vi "MESS压力值上传测试.vi"(8 "error in (no error)":errorcluster caption="错误输入（无错误）", 9 "barcode":string="C0C50E0004010", 10 "accessKey":string="a45b2d3334ffs_", 11 "Url":string="http://10.6.1.31:8080/MesInnerpackLineIO.asmx") -> (0 "error out":errorcluster caption="错误输出", 3 "ValidateBarcode":string="True,10270194,C.0C.50E,Firehawk药物支架系统（CE无标签）RV3035,RV3035,10")   [LabVIEW 2017]
uses:
  D:/Inspect System/Source Code/Andafa.IO.Helper.dll
  Andafa.IO.Helper.dll
panel:
  # "http://10.6.1.31:8080/MesInnerpackLineIO.asmx"
  # "a45b2d3334ffs_"
  # "C0C50E0004010"
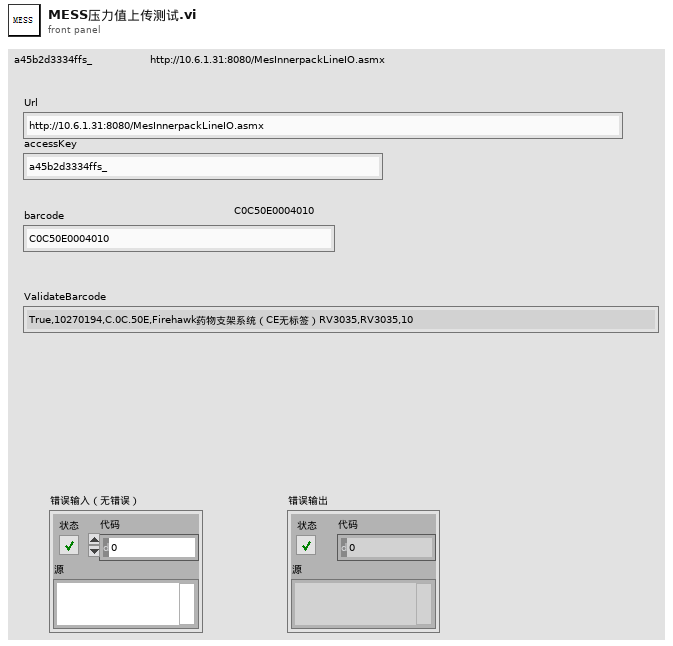
[diagram p1: front panel]
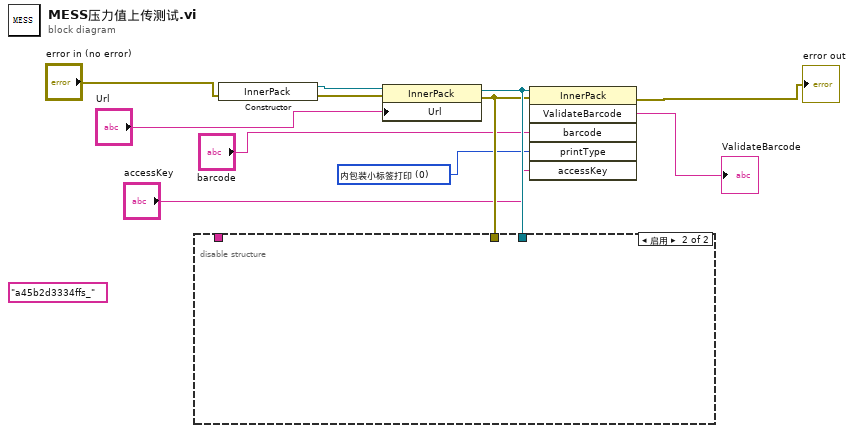
[diagram p0: block diagram]
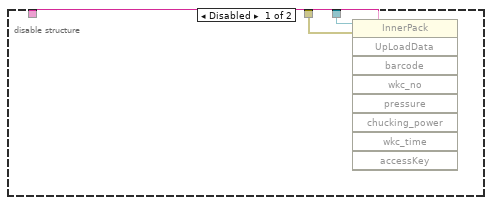
[diagram p2: hidden frame]
diagram:
  (unwired) "a45b2d3334ffs_" ("accessKey")
  w3 = 0 items=["内包装小标签打印", "内包装小标签补打"] ("printType")
  n1 = constructor class="InnerPack"(error in="error in (no error)") -> (reference out=w11:refnum<k24>, error out=w10:errorcluster)  [unwired: 2 in, 1 out]
  n2 = property on="属性节点" class="InnerPack"(reference=w11, error in=w10, "Url"="Url") -> (reference out=w7:refnum<k24>, error out=w6:errorcluster)
  n3 = disable-structure shown="启用" {
    disable-tunnel: w7 -> [w14 _]
    disable-tunnel: w6 -> [w13 _]
    disable-tunnel: _ -> [w12 _]
    frame Disabled {
      n4 = invoke on="调用节点" class="InnerPack" method="UpLoadData"(reference=w14, error in=w13, "accessKey"=w12) -> ()  [unwired: 6 in, 9 out]
    }
    frame Enabled {
    }
  }
  n5 = invoke on="调用节点" class="InnerPack" method="ValidateBarcode"(reference=w7, error in=w6, "barcode"="barcode", "printType"=w3, "accessKey"="accessKey") -> (error out=→"error out":errorcluster, "ValidateBarcode"=→"ValidateBarcode":string)  [unwired: 1 in, 4 out]
